vi "linear_ramp_with_sinusoidal_return_and_phase_shift.vi"(7 "Sweep Interval (µS)":u32, 8 "Offset":dbl, 9 "Amplitude":dbl, 10 "Phase Shift (µs)":i32, 11 "Sweep Time (µs)":u32) -> (1 "Waveform Chart":waveform(dbl)(graph))   [LabVIEW 2012]
uses:
  <vilib>/Analysis/1siggen.llb/Ramp Pattern by Samples.vi
  <vilib>/Analysis/NI_AALBase.lvlib
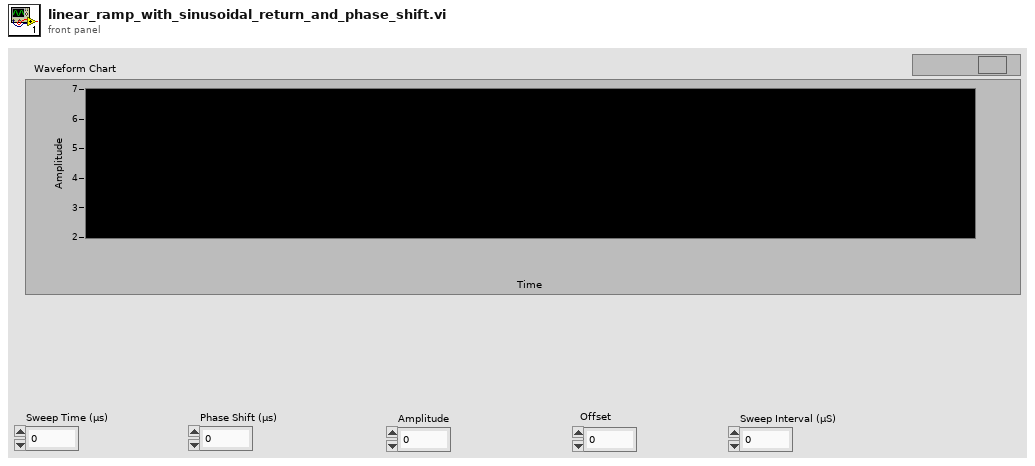
[diagram p1: front panel]
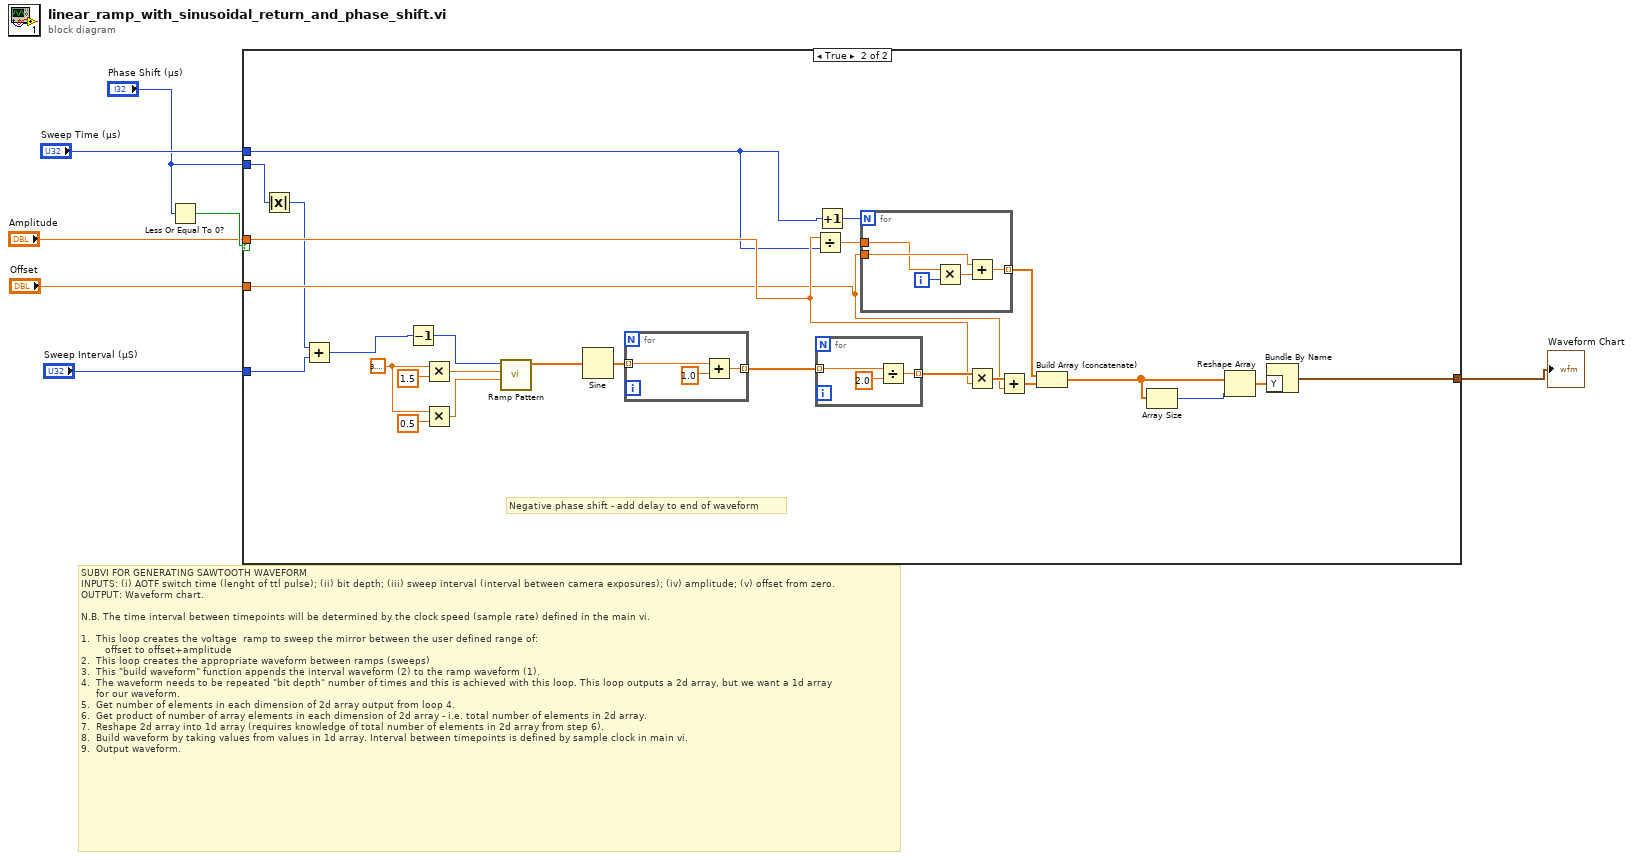
[diagram p0: block diagram]
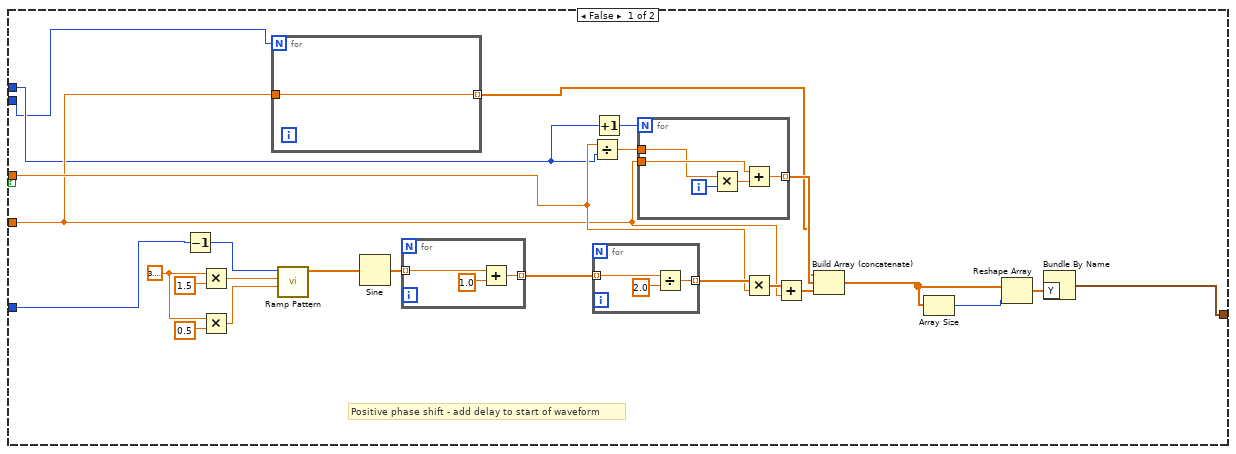
[diagram p2: hidden frame]
diagram:
  # "SUBVI FOR GENERATING SAWTOOTH WAVEFORM\nINPUTS: (i) AOTF switch time (lenght of ttl pulse); (ii) bit depth; (iii) sweep interval (interval between camera exposures); (iv) amplitude; (v) offset from zero.\nOUTPUT: Waveform chart.\n\nN.B. The time interval between timepoints will be determined by the clock speed (sample rate) defined in the main vi. \n\n1.  This loop creates the voltage  ramp to sweep the mirror between the user defined range of: \n        offset to offset+amplitude\n2.  This loop creates the appropriate waveform between ramps (sweeps)\n3.  This \"build waveform\" function appends the interval waveform (2) to the ramp waveform (1).\n4.  The waveform needs to be repeated \"bit depth\" number of times and this is achieved with this loop. This loop outputs a 2d array, but we want a 1d array \n     for our waveform.\n5.  Get number of elements in each dimension of 2d array output from loop 4.\n6.  Get product of number of array elements in each dimension of 2d array - i.e. total number of elements in 2d array.\n7.  Reshape 2d array into 1d array (requires knowledge of total number of elements in 2d array from step 6).\n8.  Build waveform by taking values from values in 1d array. Interval between timepoints is defined by sample clock in main vi.\n9.  Output waveform."
  n1 = Less Or Equal To 0?(x="Phase Shift (µs)") -> (x <= 0?=w6:bool)
  n2 = case shown="True" w6 {
    tunnel: [w14 w52] -> w7
    tunnel: "Sweep Time (µs)" -> [w10 w47]
    tunnel: "Amplitude" -> [w13 w51]
    tunnel: "Offset" -> [w11 w50]
    tunnel: "Sweep Interval (µS)" -> [w8 w49]
    tunnel: "Phase Shift (µs)" -> [w9 w46]
    frame False {
      w19 = 3.141592653589793
      # "Positive phase shift - add delay to start of waveform"
      n3 = Decrement(x=w8) -> (x-1=w29:u32)
      n4 = Multiply(x=w19, y=1.5) -> (x*y=w23:dbl)
      n5 = Multiply(x=w19, y=0.5) -> (x*y=w22:dbl)
      n6 = for {
        N: w9 -> [_]
        tunnel: [w33] -> w12 mode=indexing
        tunnel: w11 -> [w33]
      }
      n7 = call-poly <vilib>:"Ramp Pattern.vi"("start"=w22, "end"=w23, "samples"=w29) -> ("Ramp Pattern"=w24:dbl[])  [unwired: 7 in, 1 out]
      n8 = Sine(x=w24) -> (sin(x)=w26:dbl[])
      n9 = for {
        tunnel: w26 -> [w39] mode=indexing
        tunnel: [w38] -> w27 mode=indexing
        n10 = Add(x=w39, y=1.0) -> (x+y=w38:dbl)
      }
      n11 = Divide(x=w13, y=w10) -> (x/y=w15:dbl)
      n12 = for {
        tunnel: w27 -> [w36] mode=indexing
        tunnel: [w35] -> w28 mode=indexing
        n13 = Divide(x=w36, y=2.0) -> (x/y=w35:dbl)
      }
      n14 = Increment(x=w10) -> (x+1=w17:u32)
      n15 = for {
        N: w17 -> [_]
        tunnel: w11 -> [w44]
        tunnel: w15 -> [w42]
        tunnel: [w40] -> w16 mode=indexing
        i -> [w43]
        n16 = Multiply(x=w42, y=w43) -> (x*y=w41:dbl)
        n17 = Add(x=w44, y=w41) -> (x+y=w40:dbl)
      }
      n18 = Multiply(x=w28, y=w13) -> (x*y=w25:dbl[])
      n19 = Add(x=w25, y=w11) -> (x+y=w30:dbl[])
      n20 = Build Array (concatenate)(w12, w16, w30) -> (w31:dbl[])
      n21 = Array Size(array=w31) -> (size(s)=w32:i32)
      n22 = Reshape Array(w31, w32) -> (w18:dbl[])
      n23 = Bundle By Name("Y"=w18) -> (w14:waveform(dbl))  [unwired: 1 in]
    }
    frame True {
      w57 = 3.141592653589793
      # "Negative phase shift - add delay to end of waveform"
      n24 = Absolute Value(x=w46) -> (abs(x)=w45:i32)
      n25 = Add(x=w45, y=w49) -> (x+y=w48:u32)
      n26 = Decrement(x=w48) -> (x-1=w67:u32)
      n27 = Multiply(x=w57, y=1.5) -> (x*y=w61:dbl)
      n28 = Multiply(x=w57, y=0.5) -> (x*y=w60:dbl)
      n29 = call-poly <vilib>:"Ramp Pattern.vi"("start"=w60, "end"=w61, "samples"=w67) -> ("Ramp Pattern"=w62:dbl[])  [unwired: 7 in, 1 out]
      n30 = Sine(x=w62) -> (sin(x)=w64:dbl[])
      n31 = for {
        tunnel: w64 -> [w76] mode=indexing
        tunnel: [w75] -> w65 mode=indexing
        n32 = Add(x=w76, y=1.0) -> (x+y=w75:dbl)
      }
      n33 = Divide(x=w51, y=w47) -> (x/y=w53:dbl)
      n34 = for {
        tunnel: w65 -> [w73] mode=indexing
        tunnel: [w72] -> w66 mode=indexing
        n35 = Divide(x=w73, y=2.0) -> (x/y=w72:dbl)
      }
      n36 = Increment(x=w47) -> (x+1=w55:u32)
      n37 = for {
        N: w55 -> [_]
        tunnel: w50 -> [w81]
        tunnel: w53 -> [w79]
        tunnel: [w77] -> w54 mode=indexing
        i -> [w80]
        n38 = Multiply(x=w79, y=w80) -> (x*y=w78:dbl)
        n39 = Add(x=w81, y=w78) -> (x+y=w77:dbl)
      }
      n40 = Multiply(x=w66, y=w51) -> (x*y=w63:dbl[])
      n41 = Add(x=w63, y=w50) -> (x+y=w68:dbl[])
      n42 = Build Array (concatenate)(w54, w68) -> (w69:dbl[])
      n43 = Array Size(array=w69) -> (size(s)=w70:i32)
      n44 = Reshape Array(w69, w70) -> (w56:dbl[])
      n45 = Bundle By Name("Y"=w56) -> (w52:waveform(dbl))  [unwired: 1 in]
    }
  }
  "Waveform Chart" <- w7
